vi "MSScript_Format_PhaseScan.vi"(9 "ValueArray":string[](array[string]), 10 "TagArray":string[](array[string]), 11 "MSScript in":refnum<class "MSScript.lvclass">) -> (0 "ValueErrorArray":bool[](array[boolean]), 1 "TagErrorArray":bool[](array[boolean]), 2 "ParamErrorArray":bool[](array[boolean]), 3 "Data":variant, 4 "#ofParamError":bool, 6 "Warning?":bool)   [LabVIEW 2018, in "MSScript.lvclass"]
uses:
  MSScript.lvclass
  Ctl/MSEditorParam phaseScan.ctl
  MSScript_Transform_UInt.vi
  MSScript_Transform_Extended.vi
  MSScript_Transform_EXTArray.vi
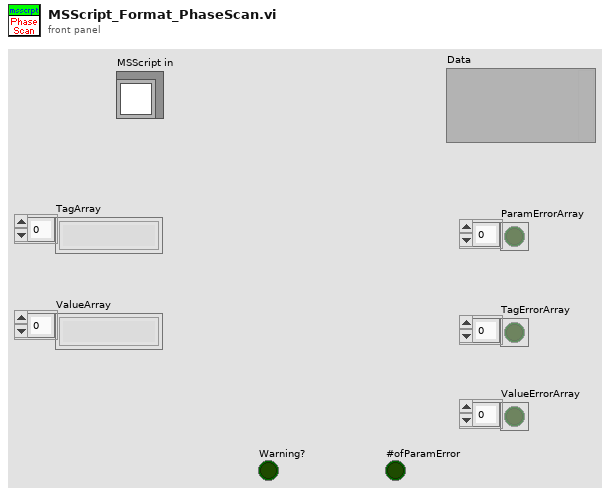
[diagram p1: front panel]
types:
  T1 = typedef "MSEditorParam phaseScan.ctl" = cluster{"auxWfmType":u32, "auxStart":u32, "iauxCyc":ext, "auxCyc":ext, "beta":ext, "betaScale":ext, "auxAmp":ext, "auxPulse1":ext[], "auxPulse2":ext[], "auxPulseAmp":ext[], "time":ext, "freq":ext[], "stepWidth":u32}
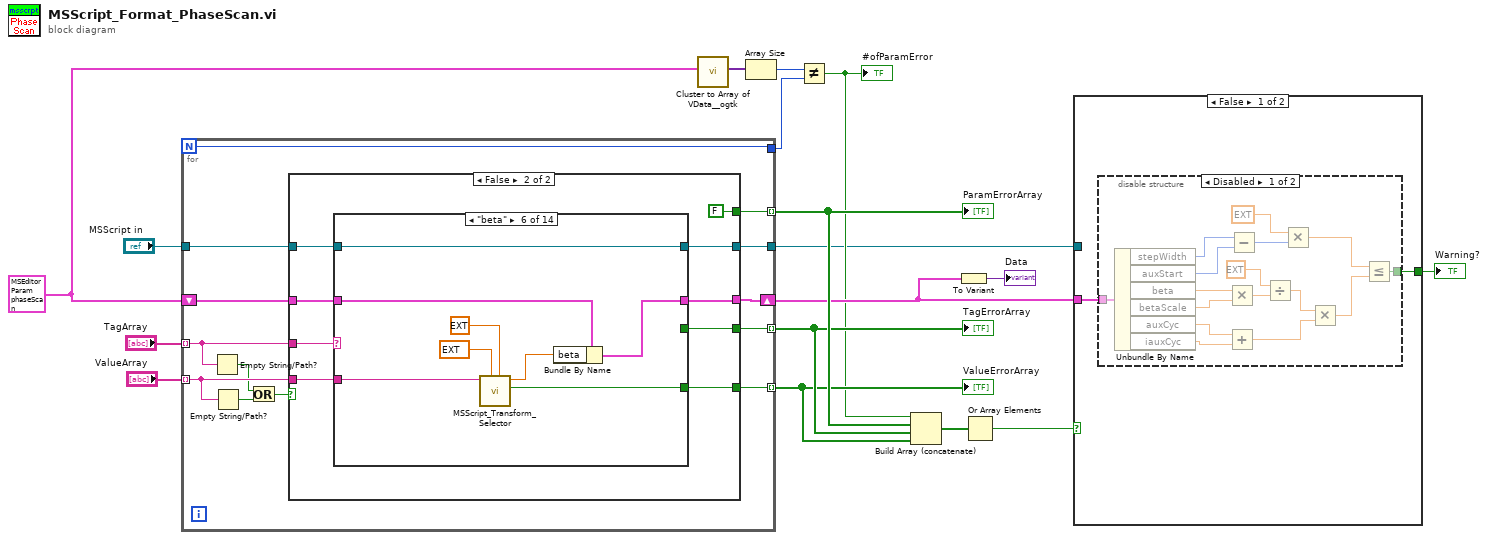
[diagram p0: block diagram]
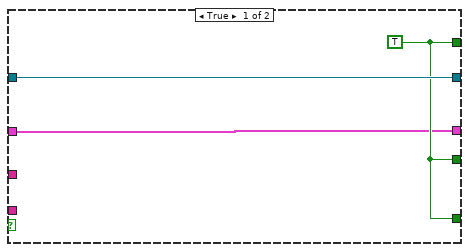
[diagram p4: hidden frame]
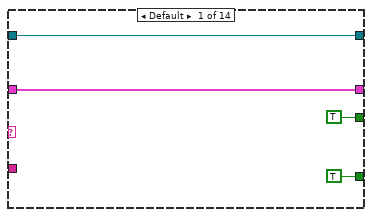
[diagram p5: hidden frame]
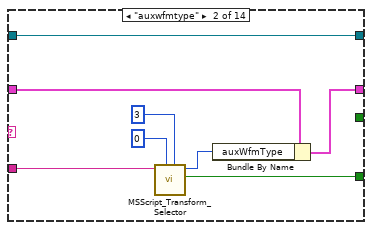
[diagram p6: hidden frame]
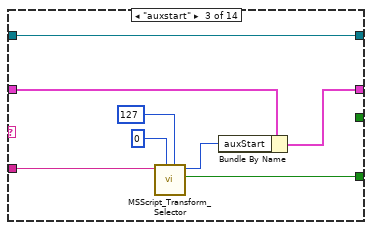
[diagram p7: hidden frame]
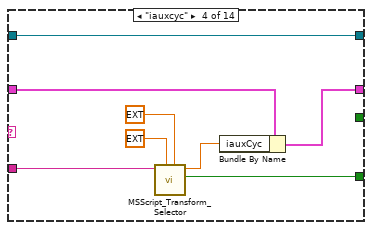
[diagram p8: hidden frame]
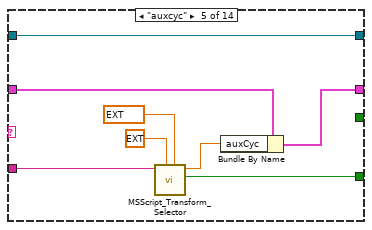
[diagram p9: hidden frame]
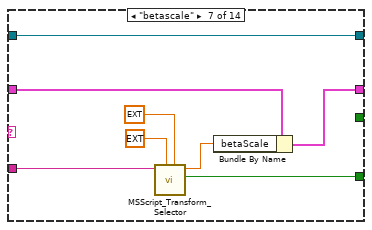
[diagram p10: hidden frame]
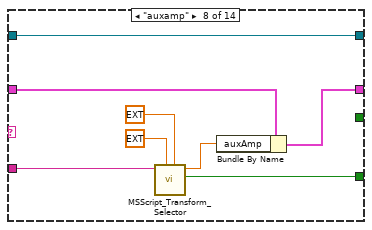
[diagram p11: hidden frame]
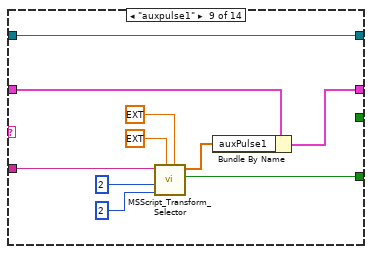
[diagram p12: hidden frame]
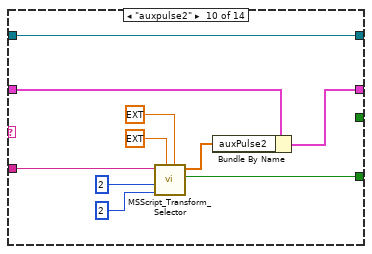
[diagram p13: hidden frame]
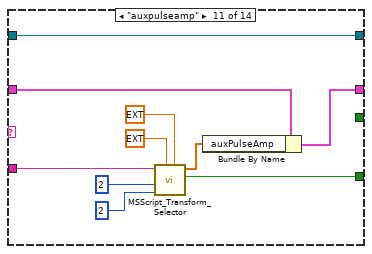
[diagram p14: hidden frame]
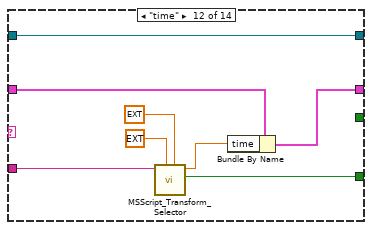
[diagram p15: hidden frame]
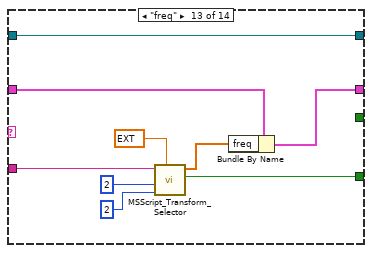
[diagram p16: hidden frame]
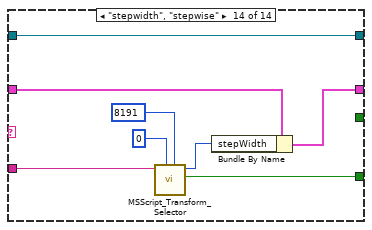
[diagram p17: hidden frame]
diagram:
  w12 = T1 {"auxWfmType"=0, "auxStart"=0, "iauxCyc"=0.0, "auxCyc"=0.0, "beta"=0.5, "betaScale"=1.0, "auxAmp"=1.0, "auxPulse1"=[0.0, 0.5], "auxPulse2"=[0.5, 1.0], "auxPulseAmp"=[1.0, -1.0], "time"=1.0, "freq"=[100000.0, 50000.0], "stepWidth"=1} ("ParamValueType")
  n1 = for {
    N -> [w18]
    tunnel: "TagArray" -> [w26] mode=indexing
    tunnel: "ValueArray" -> [w25] mode=indexing
    tunnel: [w30] -> w8 mode=indexing
    tunnel: "MSScript in" -> [w29]
    tunnel: [w28] -> w7 mode=indexing
    tunnel: [w27] -> w1
    tunnel: [w21] -> w9 mode=indexing
    shift-right: [w19] -> w4
    shift-left: w12 -> [w20]
    tunnel: [w18] -> w11
    n2 = Empty String/Path?(string/path=w26) -> (empty?=w23:bool)
    n3 = Empty String/Path?(string/path=w25) -> (empty?=w24:bool)
    n4 = Or(x=w23, y=w24) -> (x .or. y?=w22:bool)
    n5 = case shown="False" w22 {
      tunnel: [w32 w35] -> w30
      tunnel: w29 -> [w33 w41]
      tunnel: [w32 w34] -> w28
      tunnel: [w33 w37] -> w27
      tunnel: w26 -> [_ w39]
      tunnel: w25 -> [_ w38]
      tunnel: [w32 FALSE] -> w21
      tunnel: w20 -> [w31 w40]
      tunnel: [w31 w36] -> w19
      frame True {
        w32 = TRUE
      }
      frame False {
        n6 = case shown="\"beta\"" w39 {
          tunnel: [TRUE _ _ _ _ _ _ _ _ _ _ _ _ _] -> w35
          tunnel: w41 -> [w44 w52 w60 w68 w76 w84 w92 w100 w110 w120 w130 w138 w143 w152]
          tunnel: w38 -> [_ w53 w61 w69 w77 w85 w93 w101 w111 w121 w131 w139 w148 w156]
          tunnel: [TRUE ("Value Error?") w54 w62 w70 w78 w86 w94 w102 w112 w122 w132 w140 w149 w157] -> w34
          tunnel: [w44 w52 w60 w68 w76 w84 w92 w100 w110 w120 w130 w138 w143 w152] -> w37
          tunnel: w40 -> [w43 w50 w58 w66 w74 w82 w90 w98 w108 w118 w128 w136 w146 w154]
          tunnel: [w43 w49 w57 w65 w73 w81 w89 w97 w107 w117 w127 w135 w145 w153] -> w36
          frame Default {
          }
          frame "auxwfmtype" {
            n7 = call-poly "MSScript_Transform_Selector.vi"("upper limit"=u64 3, "lower limit"=u64 0, "string in"=w53) -> ("Value Error?"=w54:bool, "Value Output"=w51:u64)  [unwired: 6 in, 1 out]
            n8 = Bundle By Name(cluster=w50, "auxWfmType"=w51) -> (w49:T1)
          }
          frame "auxstart" {
            n9 = call-poly "MSScript_Transform_Selector.vi"("upper limit"=u64 127, "lower limit"=u64 0, "string in"=w61) -> ("Value Error?"=w62:bool, "Value Output"=w59:u64)  [unwired: 6 in, 1 out]
            n10 = Bundle By Name(cluster=w58, "auxStart"=w59) -> (w57:T1)
          }
          frame "iauxcyc" {
            n11 = call-poly "MSScript_Transform_Selector.vi"("upper limit (Inf)"=ext 1.0 ("upper limit"), "lower limit (-Inf)"=ext 0.0 ("lower limit"), "Check_Str"=w69) -> ("Value Error?"=w70:bool, "Value Output"=w67:ext)  [unwired: 6 in, 1 out]
            n12 = Bundle By Name(cluster=w66, "iauxCyc"=w67) -> (w65:T1)
          }
          frame "auxcyc" {
            n13 = call-poly "MSScript_Transform_Selector.vi"("upper limit (Inf)"=ext 99999.0 ("upper limit"), "lower limit (-Inf)"=ext 0.0 ("lower limit"), "Check_Str"=w77) -> ("Value Error?"=w78:bool, "Value Output"=w75:ext)  [unwired: 6 in, 1 out]
            n14 = Bundle By Name(cluster=w74, "auxCyc"=w75) -> (w73:T1)
          }
          frame "beta" {
            n15 = call-poly "MSScript_Transform_Selector.vi"("upper limit (Inf)"=ext 1.0 ("upper limit"), "lower limit (-Inf)"=ext 0.01 ("lower limit"), "Check_Str"=w85) -> ("Value Error?"=w86:bool, "Value Output"=w83:ext)  [unwired: 6 in, 1 out]
            n16 = Bundle By Name(cluster=w82, "beta"=w83) -> (w81:T1)
          }
          frame "betascale" {
            n17 = call-poly "MSScript_Transform_Selector.vi"("upper limit (Inf)"=ext 10.0 ("upper limit"), "lower limit (-Inf)"=ext 0.0 ("lower limit"), "Check_Str"=w93) -> ("Value Error?"=w94:bool, "Value Output"=w91:ext)  [unwired: 6 in, 1 out]
            n18 = Bundle By Name(cluster=w90, "betaScale"=w91) -> (w89:T1)
          }
          frame "auxamp" {
            n19 = call-poly "MSScript_Transform_Selector.vi"("upper limit (Inf)"=ext 1.0 ("upper limit"), "lower limit (-Inf)"=ext 0.0 ("lower limit"), "Check_Str"=w101) -> ("Value Error?"=w102:bool, "Value Output"=w99:ext)  [unwired: 6 in, 1 out]
            n20 = Bundle By Name(cluster=w98, "auxAmp"=w99) -> (w97:T1)
          }
          frame "auxpulse1" {
            n21 = call-poly "MSScript_Transform_Selector.vi"("upper limit (Inf)"=ext 1.0 ("upper limit"), "lower limit (-Inf)"=ext 0.0 ("lower limit"), "MinSize"=u8 2 ("MaxSize"), "MaxSize"=u8 2, "check_str"=w111) -> ("Value Error?"=w112:bool, "Value Output"=w109:ext[])  [unwired: 4 in, 1 out]
            n22 = Bundle By Name(cluster=w108, "auxPulse1"=w109) -> (w107:T1)
          }
          frame "auxpulse2" {
            n23 = call-poly "MSScript_Transform_Selector.vi"("upper limit (Inf)"=ext 1.0 ("upper limit"), "lower limit (-Inf)"=ext 0.0 ("lower limit"), "MinSize"=u8 2 ("MaxSize"), "MaxSize"=u8 2, "check_str"=w121) -> ("Value Error?"=w122:bool, "Value Output"=w119:ext[])  [unwired: 4 in, 1 out]
            n24 = Bundle By Name(cluster=w118, "auxPulse2"=w119) -> (w117:T1)
          }
          frame "auxpulseamp" {
            n25 = call-poly "MSScript_Transform_Selector.vi"("upper limit (Inf)"=ext 1.0 ("upper limit"), "lower limit (-Inf)"=ext -1.0 ("lower limit"), "MinSize"=u8 2 ("MaxSize"), "MaxSize"=u8 2, "check_str"=w131) -> ("Value Error?"=w132:bool, "Value Output"=w129:ext[])  [unwired: 4 in, 1 out]
            n26 = Bundle By Name(cluster=w128, "auxPulseAmp"=w129) -> (w127:T1)
          }
          frame "time" {
            n27 = call-poly "MSScript_Transform_Selector.vi"("upper limit (Inf)"=ext 60.0 ("upper limit"), "lower limit (-Inf)"=ext 0.0 ("lower limit"), "Check_Str"=w139) -> ("Value Error?"=w140:bool, "Value Output"=w137:ext)  [unwired: 6 in, 1 out]
            n28 = Bundle By Name(cluster=w136, "time"=w137) -> (w135:T1)
          }
          frame "freq" {
            n29 = call-poly "MSScript_Transform_Selector.vi"("lower limit (-Inf)"=ext 0.01 ("lower limit"), "MinSize"=u8 2 ("MaxSize"), "MaxSize"=u8 2, "check_str"=w148) -> ("Value Error?"=w149:bool, "Value Output"=w147:ext[])  [unwired: 5 in, 1 out]
            n30 = Bundle By Name(cluster=w146, "freq"=w147) -> (w145:T1)
          }
          frame "stepwidth", "stepwise" {
            n31 = call-poly "MSScript_Transform_Selector.vi"("upper limit"=u64 8191, "lower limit"=u64 0, "string in"=w156) -> ("Value Error?"=w157:bool, "Value Output"=w155:u64)  [unwired: 6 in, 1 out]
            n32 = Bundle By Name(cluster=w154, "stepWidth"=w155) -> (w153:T1)
          }
        }
      }
    }
  }
  "TagErrorArray" <- w8
  "ValueErrorArray" <- w7
  "ParamErrorArray" <- w9
  n33 = call <userlib>:"Cluster to Array of VData__ogtk.vi"("Cluster"=w12) -> ("Array of VData"=w14:variant[])  [unwired: 9 in, 1 out]
  n34 = Array Size(array=w14) -> (size(s)=w13:i32)
  n35 = Not Equal?(x=w13, y=w11) -> (x != y?=w2:bool)
  "#ofParamError" <- w2
  n36 = Build Array (concatenate)(w2, w9, w8, w7) -> (w6:bool[])
  n37 = To Variant(anything=w4) -> (Variant=→"Data":variant)
  n38 = Or Array Elements(Boolean array=w6) -> (logical OR=w5:bool)
  n39 = case shown="False" w5 {
    tunnel: w4 -> [w159 _]
    tunnel: [w158 _] -> w3
    tunnel: w1 -> [_ _]
    frame False {
      n40 = disable-structure shown="Disabled" {
        disable-tunnel: w159 -> [w175 _]
        disable-tunnel: [w160 _] -> w158
        frame Disabled {
          n41 = Unbundle By Name(w175) -> ("stepWidth"=w174:u32, "auxStart"=w173:u32, "beta"=w169:ext, "betaScale"=w168:ext, "auxCyc"=w165:ext, "iauxCyc"=w164:ext)
          n42 = Multiply(x=w169, y=w168) -> (x*y=w166:ext)
          n43 = Add(x=w165, y=w164) -> (x+y=w163:ext)
          n44 = Subtract(x=w174, y=w173) -> (x-y=w171:u32)
          n45 = Divide(x=ext 2.0, y=w166) -> (x/y=w162:ext)
          n46 = Multiply(x=ext 0.5, y=w171) -> (x*y=w170:ext)
          n47 = Multiply(x=w162, y=w163) -> (x*y=w161:ext)
          n48 = Less Or Equal?(x=w170, y=w161) -> (x <= y?=w160:bool)
        }
        frame Enabled {
        }
      }
    }
    frame True {
    }
  }
  "Warning?" <- w3
